vi "Display Console - Init.vi"(8 "error in (no error)":errorcluster, 11 "GUI Refs":T1) -> (0 "error out":errorcluster)   [LabVIEW 2017]
doc: "Initialize all GUI elevents of Display Console"
uses:
  Controls/Display Console - GUI refs.ctl
  Controller/Controls/Elevator Location.ctl
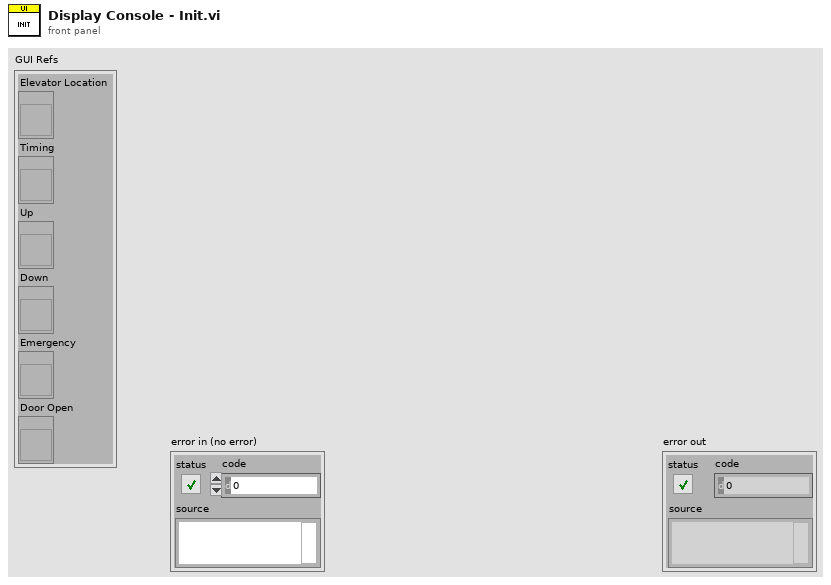
[diagram p1: front panel]
types:
  T1 = typedef "Display Console - GUI refs.ctl" = cluster{"Elevator Location":refnum<vi>, "Timing":refnum<vi>, "Up":refnum<vi>, "Down":refnum<vi>, "Emergency":refnum<vi>, "Door Open":refnum<vi>}
  T2 = typedef "Elevator Location.ctl" = enum16{"1st Floor", "2nd Floor", "3rd Floor", "4th Floor"}
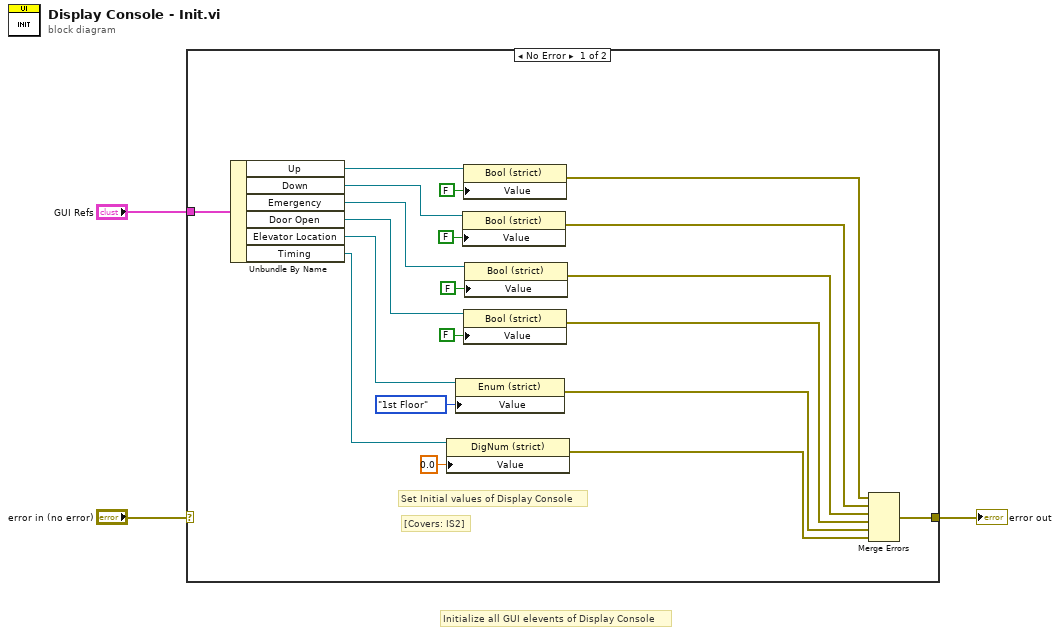
[diagram p0: block diagram]
diagram:
  # "Initialize all GUI elevents of Display Console"
  n1 = case shown="No Error" "error in (no error)" {
    selector: "error in (no error)" -> [_ w24]
    tunnel: [w20 w24] -> w2
    tunnel: "GUI Refs" -> [w23 _]
    frame No Error {
      # "[Covers: IS2]"
      # "Set Initial values of Display Console"
      n2 = Unbundle By Name(w23) -> ("Up"=w22:refnum<vi>, "Down"=w18:refnum<vi>, "Emergency"=w13:refnum<vi>, "Door Open"=w12:refnum<vi>, "Elevator Location"=w11:refnum<vi>, "Timing"=w10:refnum<vi>)
      n3 = property class="DigNum (strict)"(reference=w10, "Value"=0.0) -> (error out=w4:errorcluster)  [unwired: 1 in, 1 out]
      n4 = property class="Enum (strict)"(reference=w11, "Value"=Elevator_Location."1st Floor") -> (error out=w5:errorcluster)  [unwired: 1 in, 1 out]
      n5 = property class="Bool (strict)"(reference=w18, "Value"=FALSE) -> (error out=w16:errorcluster)  [unwired: 1 in, 1 out]
      n6 = property class="Bool (strict)"(reference=w22, "Value"=FALSE) -> (error out=w17:errorcluster)  [unwired: 1 in, 1 out]
      n7 = property class="Bool (strict)"(reference=w12, "Value"=FALSE) -> (error out=w6:errorcluster)  [unwired: 1 in, 1 out]
      n8 = property class="Bool (strict)"(reference=w13, "Value"=FALSE) -> (error out=w7:errorcluster)  [unwired: 1 in, 1 out]
      n9 = Merge Errors(w17, w16, w7, w6, w5, w4) -> (w20:errorcluster)
    }
    frame Error {
    }
  }
  "error out" <- w2
